vi "MLS_Read_subVI.vi"(2 "Filename":string="MLS.txt", 3 "Amplitude":dbl=2.0) -> (0 "Path":path, 1 "Waveform Graph":dbl[](graph))   [LabVIEW 2016]
uses:
  <vilib>/Utility/file.llb/Read Delimited Spreadsheet (DBL).vi
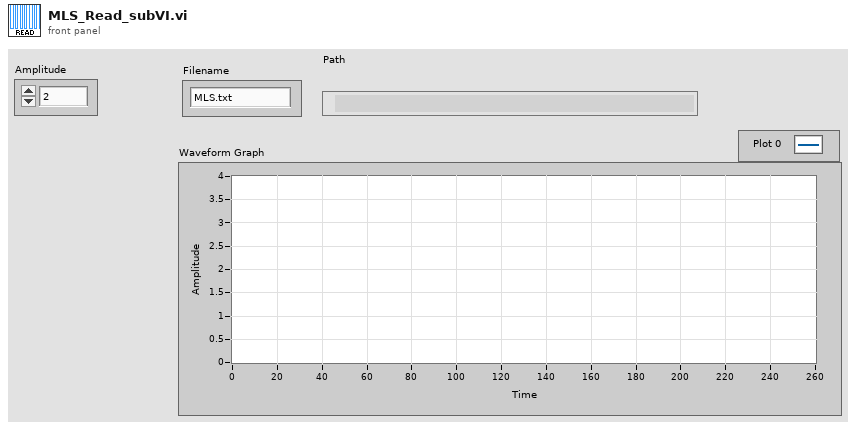
[diagram p1: front panel]
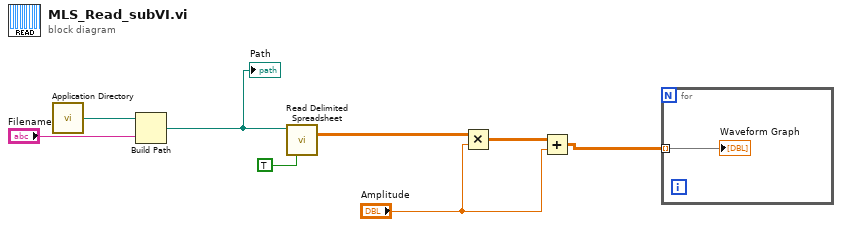
[diagram p0: block diagram]
diagram:
  n1 = call <vilib>:"Application Directory.vi"() -> ("Application Directory"=w7:path)
  n2 = Build Path(base path=w7, name or relative path="Filename") -> (appended path=w6:path)
  "Path" <- w6
  n3 = call-poly <vilib>:"Read Delimited Spreadsheet.vi"("file path (dialog if empty)"=w6, "transpose? (F)"=TRUE) -> ("all rows"=w2:dbl[][])  [unwired: 8 in, 5 out]
  n4 = Multiply(x=w2, y="Amplitude") -> (x*y=w5:dbl[][])
  n5 = Add(x=w5, y="Amplitude") -> (x+y=w1:dbl[][])
  n6 = for {
    tunnel: w1 -> [w9] mode=indexing
    "Waveform Graph" <- w9
  }
